vi "Get History All.vi"(8 "error in (no error)":errorcluster, 11 "BME280 in":refnum<class "BME280.lvclass">) -> (0 "error out":errorcluster, 3 "BME280 out":refnum<class "BME280.lvclass">)   [LabVIEW 2020, in "BME280.lvclass"]
uses:
  BME280.lvclass
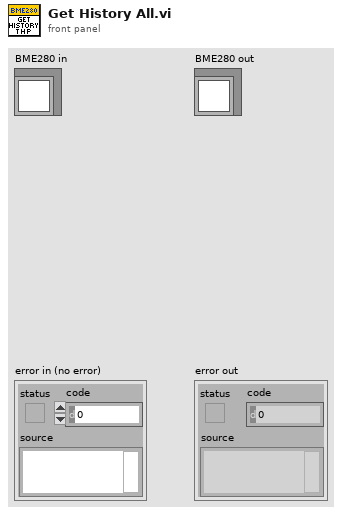
[diagram p1: front panel]
types:
  T1 = typedef "BME280.lvclass/Weather.ctl" = cluster{"temperature":dbl[], "humidity":dbl[], "pressure":dbl[]}
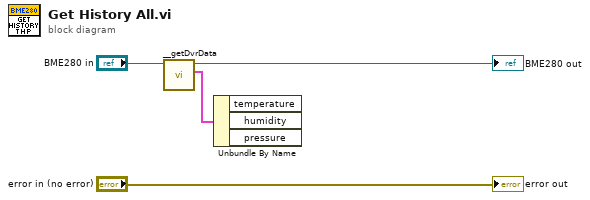
[diagram p0: block diagram]
diagram:
  n1 = call "__getDvrData.vi"("BME280 in"="BME280 in") -> ("weather"=w2:T1, "BME280 out"=→"BME280 out":refnum<class "BME280.lvclass">)  [unwired: 8 in, 1 out]
  n2 = Unbundle By Name(w2) -> ()  [unwired: 3 out]
  "error out" <- "error in (no error)"
